vi "qSTV.vi"(0 "System no.":i32=1 min=1 max=4 step=1, 2 "Status Type":string[](array[string]), 5 "error in":errorcluster) -> (14 "Status Array":T1[](array[typedef]), 19 "error out":errorcluster)   [LabVIEW 2026]
doc: "GCS 3.0\n=====\n\nSTV? (Query Status Values) \n\nDescription\nReads out the status register of a container unit (p. 91). \n\nFormat\nSTV?[ <Container Unit>]\n\nArguments\n<Container Unit>\nContainer unit, deren Statusregister abgefragt werden sollDie Container Units, für die ein \nStatusregister vorhanden ist, können mit USG? CMD STV? abgefragt werden. Aktuell haben nur \ndie Container-Unit-Familien \"Axis\" und \"System\" Statusregister.\nPossible values: Alias of the container unit (p. 94) \n\nResponse\n{<Container Unit>\"=\"<Value>LF}\n<Value> shows the state of the container unit. The 32-bit value is bit coded and is output in the \nhexadecimal format.\n\nExample\nThere is no motion error for axis 1. Drive and control are switched on. The control variable is \nthe position. The target position has been reached. \n>>eax? axis_1\n<<AXIS_1=1\n>>sam? axis_1\n<<AXIS_1=0x2\n>>stv? axis_1\n<<AXIS_1=0x202A\n\nNotes\nThe RES command (p. 51) resets the bit for the motion error in the status register of the axis\n(p. 97). \nA query with LOG? (p. 21) resets the bits for errors from the classes Critical, Info, and Warning \nin the status register of the system (p. 99). \nThe bit for errors of the Command class is reset in the status register of the system with the \nERR? command (p. 13). \n\nUser command level\nUSR\n\n\nGCS 2.0\n=====\n\nSTV? (Query Status Values)\n\nSystem Status\n0 Command Error\n1 Critical Error\n2 Information\n3 Warning\n\n\nAxis Status bit\n0 Error\n1 EAX? (axis enabled)\n2 FBA (active error handling)\n3 OL/CL controller enabled\n4-11 MOP Bit 0-7\n12 FRF?\n13 ONT?\n14 IPR\n15 PLim\n16 NLim\n17 Ref\n18 In motion"
uses:
  Status.ctl
panel:
  # "STV? (Query Status Values) \n\nReads out the status register of a container unit."
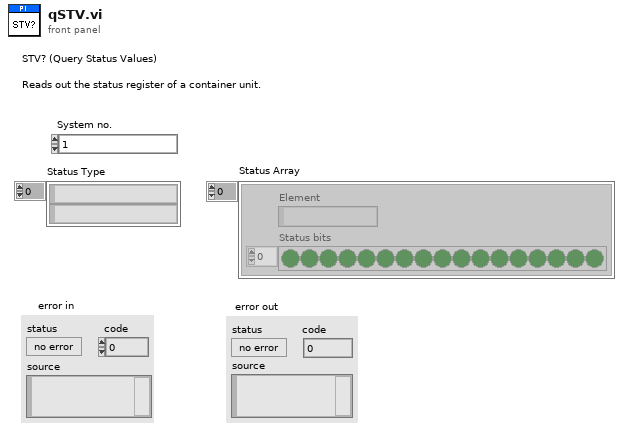
[diagram p1: front panel]
types:
  T1 = typedef "Status.ctl" = cluster{"Element":string, "Status bits":bool[]}
  T2 = typedef "Syntax.ctl" = enum16{"GCS 1.0", "GCS 2.0", "GCS 3.0"}
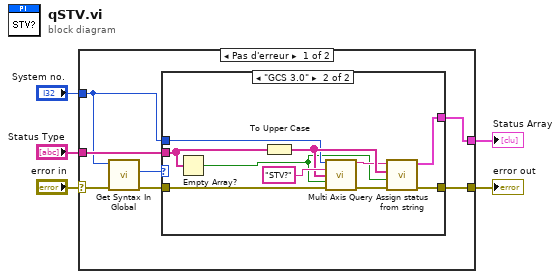
[diagram p0: block diagram]
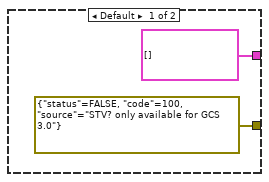
[diagram p2: hidden frame]
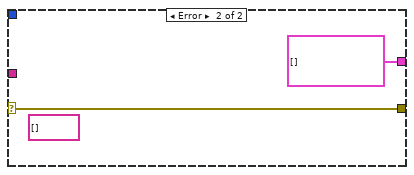
[diagram p3: hidden frame]
diagram:
  n1 = case shown="Pas d'erreur" "error in" {
    selector: "error in" -> [w9 w26]
    tunnel: "Status Type" -> [w12 _]
    tunnel: [w11 w26] -> w2
    tunnel: "System no." -> [w7 _]
    tunnel: [w10 T1[] [] ("Status Array")] -> w1
    frame No Error {
      n2 = call "Get Syntax In Global.vi"("error in"=w9, "System no."=w7) -> ("error out"=w8:errorcluster, "Syntax"=w6:T2)  [unwired: 8 in]
      n3 = case shown="\"GCS 3.0\"" w6 {
        tunnel: w12 -> [_ w15]
        tunnel: [errorcluster {"status"=FALSE, "code"=100, "source"="STV? only available for GCS 3.0"} ("error out") w22] -> w11
        tunnel: [T1[] [] ("Status Array") w19] -> w10
        tunnel: w8 -> [_ w18]
        tunnel: w7 -> [_ w17]
        frame Default {
        }
        frame "GCS 3.0" {
          n4 = Empty Array?(array=w15) -> (empty?=w16:bool)
          n5 = To Upper Case(1:w15) -> (0:w21:string[])
          n6 = call "Multi Axis Query.vi"("System no."=w17, "Command"="STV?", "Axis"=w21, "All axes?"=w16, "error in (no error)"=w18) -> ("Answer"=w20:string, "error out"=w23:errorcluster)  [unwired: 9 in]
          n7 = call "Assign status from string.vi"("error in (no error)"=w23, "Read All Lines?"=w16, "Elements to parse"=w21, "Answer to parse"=w20) -> ("error out"=w22:errorcluster, "Status Array"=w19:T1[])  [unwired: 6 in]
        }
      }
    }
    frame Error {
      (unwired) string[] [] ("Axes to query out")
    }
  }
  "error out" <- w2
  "Status Array" <- w1
